vi "Get License State.vi"() -> ()   [LabVIEW 2018]
doc: "Demonstrates how to get the license state of a software toolkit."
panel:
  in  "runtime":bool
  out "License State":string
  in  "product name":string(combo)="opencv_dnn"
  # "Overview: Demonstrates how to get the license state of a software toolkit.\nRequirements: Windows.\nInstructions: \n1. Fill in the product name (opencv_dnn, openvino, onnx_gpu, tensorRT and etc), and select if the toolkit is running in LabVIEW Runtime.\n2. Run the VI.\n3. This VI returns the license state corresponding to the name in the \"product_name\" control."
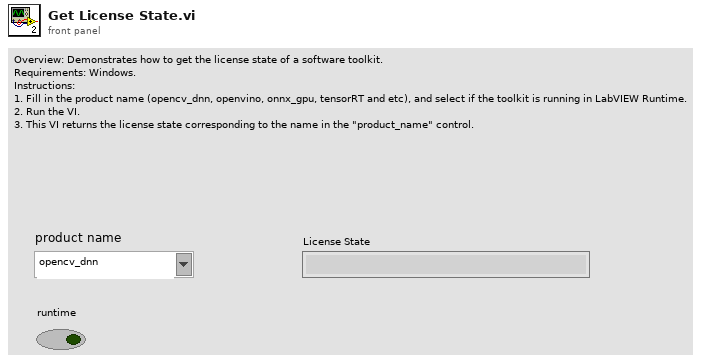
[diagram p1: front panel]
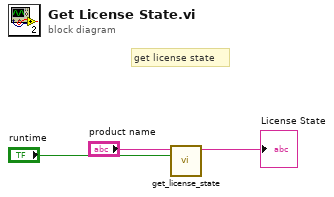
[diagram p0: block diagram]
diagram:
  # "get license state"
  n1 = call "get_license_state.vi"("runtime"="runtime", "product name"="product name") -> ("network License State"=→"License State":string)  [unwired: 8 in, 1 out]
